vi "destroy_Host.vi"(8 "error in (no error)":errorcluster, 10 "LabVIEW Object":refnum<class>, 11 "MoAgSy_Host in":refnum<class "MoAgSy_Host.lvclass">) -> (0 "error out":errorcluster)   [LabVIEW 2009, in "MoAgSy.lvlib" / "MoAgSy_Host.lvclass"]
doc: "<B>public</B> VI destroys a Host.\nWhether Labview Object or Host in can be used as input.\nAll kill occurences will be set. Threadpool and DSC will be ended.\nIf no error occurred, Host init data will be stored on disk in local working folder.\n\nF.Berck@gsi.de\nGSI Darmstadt 2009"
uses:
  MoAgSy_Host.lvclass
  HGF_BaseClasses/HGF_ThreadPool/HGF_ThreadPool.lvclass
  HGF_BaseClasses/HGF_Reference/HGF_Reference.lvclass
  HGF_BaseClasses/HGF_Factory/HGF_Factory.lvclass
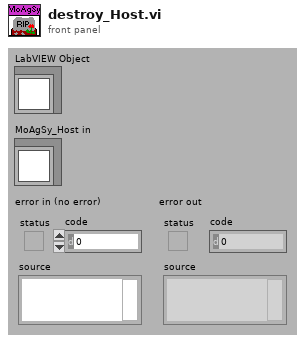
[diagram p1: front panel]
types:
  T1 = cluster{"killNotifier":refnum<notifier>, "Agent ID":string}[]
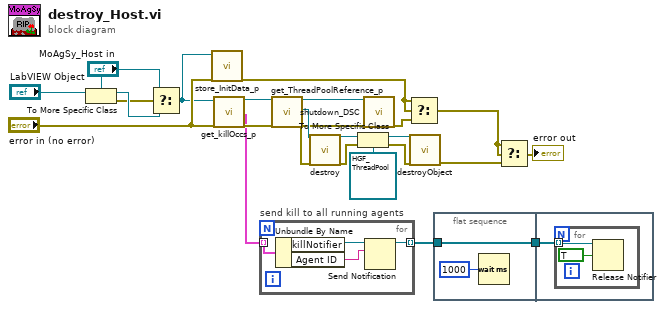
[diagram p0: block diagram]
diagram:
  n1 = To More Specific Class(target class="MoAgSy_Host in", reference="LabVIEW Object") -> (specific class reference=w23:refnum<class "MoAgSy_Host.lvclass">, error out=w13:errorcluster)  [unwired: 1 in]
  n2 = Select(t="MoAgSy_Host in", s=w13, f=w23) -> (s? t:f=w1:refnum<class "MoAgSy_Host.lvclass">)
  n3 = call "store_InitData_p.vi"("MoAgSy_Host in"=w1, "error in (no error)"="error in (no error)") -> ("error out"=w2:errorcluster)  [unwired: 17 out]
  n4 = call "get_killOccs_p.vi"("MoAgSy_Host"=w1, "error in (no error)"="error in (no error)") -> ("dup MoAgSy_Host"=w21:refnum<class "MoAgSy_Host.lvclass">, "Kill Occs"=w12:T1, "error out"=w20:errorcluster)  [unwired: 15 out]
  n5 = for "send kill to all running agents" {
    tunnel: w12 -> [w28] mode=indexing
    tunnel: [w25] -> w11 mode=indexing
    n6 = Unbundle By Name(w28) -> ("killNotifier"=w27:refnum<notifier>, "Agent ID"=w26:string)
    n7 = Send Notification(notification=w26, notifier=w27) -> (notifier out=w25:refnum<notifier>)  [unwired: 1 in, 1 out]
  }
  n8 = call "get_ThreadPoolReference_p.vi"("MoAgSy_Host"=w21, "error in (no error)"=w20) -> ("dup MoAgSy_Host"=w6:refnum<class "MoAgSy_Host.lvclass">, "Threadpool_Reference"=w19:refnum<class "HGF_Reference.lvclass">, "error out"=w7:errorcluster)  [unwired: 15 out]
  n9 = call "destroy.vi"("HGF_Reference"=w19, "error in (no error)"=w7) -> ("Object"=w17:refnum<class>, "error out"=w18:errorcluster)  [unwired: 2 in, 14 out]
  n10 = To More Specific Class(target class=refnum<class "HGF_ThreadPool.lvclass"> refnum ("HGF_BaseClasses.lvlib:HGF_ThreadPool.lvclass"), reference=w17, error in=w18) -> (specific class reference=w15:refnum<class "HGF_ThreadPool.lvclass">, error out=w14:errorcluster)
  n11 = call "shutdown_DSC.vi"("MoAgSy_Host"=w6, "error in (no error)"=w7) -> ("error out"=w4:errorcluster)  [unwired: 17 out]
  n12 = Select(t=w2, s=w2, f=w4) -> (s? t:f=w3:errorcluster)
  n13 = call "destroyObject.vi"("HGF_Factory"=w15, "error in (no error)"=w14) -> ("error out"=w8:errorcluster)  [unwired: 17 out]
  n14 = flat-sequence {
    tunnel: w11 -> [w30]
    tunnel: [w30] -> w10
    tunnel: w10 -> [w31]
    frame #0 {
      n15 = Wait (ms)(milliseconds to wait=u32 1000) -> ()  [unwired: 1 out]
    }
    frame #1 {
      n16 = for {
        tunnel: w31 -> [w33] mode=indexing
        n17 = Release Notifier(notifier=w33, force destroy? (F)=TRUE) -> ()  [unwired: 1 in, 3 out]
      }
    }
  }
  n18 = Select(t=w3, s=w3, f=w8) -> (s? t:f=→"error out":errorcluster)
